vi "LoadRIOSettings.vi"(8 "Error in":errorcluster, 10 "Current ExpState IN":T1={"error"={"status"=FALSE, "code"=0, "source"=""}, "Digitizer DAQmx Tasks"={"TaskArray"=[]}, "DAQ Settings"={"Channel Settings"=[], "Card Settings"=[]}, "Synchronization Settings"={"Synchronizer 0"="", "source terminal"="", "Synchronizer 1"=""}, "DAQ Data"=[], "Next Shot#"="", "System Message"="", "User Shot Notes"="", "Timing Settings"={"Timing Card Settings"=[], "Timing Channel Settings"=[]}, "Timing Tasks"={"TaskArray"=[]}, "Tree"="", "Time Card/Channels"=[], "DAQ Card/Channels"=[], "Program Version"="", "RIO Settings"={"Channel Settings"=[], "Card Settings"=[]}, "RIO References"={"Reference Array"=[]}, "RIO Data"={"RIO Deleaved Data"=[], "Raw Readout"=[]}, "RIO Card/Channels"=[], "DIO Channels"=0, "DIO Settings"={"DIO Channel Array"=[]}, "Tachometer Controls"={"Tach Calibration folder"=path "Z:/Data/Calibration/Tachometer", "PSU2 charging Voltage [kV]"=0.0, "PSU2 Counter"="", "PSU2 task"="PSU2", "PSU3 Counter"="", "PSU3 task"="", "PSU3 charging Voltage [kV]"=0.0}, "Global Settings"={"Initial Background Values"={"Reference Shot #"=0.0, "Background pressure [Torr]"=0.0, "Cryo temp [V]"=0.0, "Cryo temp [K]"=0.0, "Cryotemp Calibration File"=path ""}, "Gas Puffing"={"Gas A type"="N", "Gas B type"="N", "Gas C type"="N", "Gas A pressure [psi]"=0.0, "Gas B pressure [psi]"=0.0, "Gas C pressure [psi]"=0.0, "Innner Electrode"="", "Middle Electrode"="", "Outer Electrode"="", "Gas A bottle pressure [psi]"=0.0, "Gas B bottle pressure [psi]"=0.0, "Gas C bottle pressure [psi]"=0.0}, "PSU Voltages"={"Bias1 Voltage [V]"=0.0, "Bias2 Voltage [V]"=0.0, "PSU1 Voltage [V]"=0.0, "Puff-PSU1 CH1 Voltage [V]"=0.0, "Puff-PSU1 CH2 Voltage [V]"=0.0, "Puff-PSU1 CH3 Voltage [V]"=0.0}, "Scope Details"={"CH1"="", "CH2"="", "CH3"="", "CH4"="", "CH1 Ground State"="Grounded", "CH2 Ground State"="Grounded", "CH3 Ground State"="Grounded", "CH4 Ground State"="Grounded"}}, "Calibrations"={"CryoTemp"={"Comment"="", "X"=[], "Y"=[]}, "PSU2 Tach"={"Comment"="", "X"=[], "Y"=[]}, "PSU3 Tach"={"Comment"="", "X"=[], "Y"=[]}}} {"Global Settings"."Initial Background Values"."Cryo temp [K]" format="%#_4g"; "RIO Settings"."Card Settings"."Sample Rate" format="%#_3p"; "Timing Settings"."Timing Channel Settings"."FrontPanelTime" format="%.3p"; "Timing Settings"."Timing Channel Settings"."Pulse width (s)" format="%.3p"; "Timing Settings"."Timing Channel Settings"."Delay (s)" format="%.3p"; "DAQ Settings"."Card Settings"."Global Edge Type" items=["Rising"=10280, "Falling"=10171]; "DAQ Settings"."Card Settings"."Sample Rate" format="%#_3p"}, 11 "Tree DVR in":refnum<data-value>) -> (0 "Error out":errorcluster, 3 "RIO Settings":T8 {"Card Settings"."Sample Rate" format="%#_3p"})   [LabVIEW 2014]
uses:
  Controls/RIOSettingsExperimentStateCluster.ctl
  Controls/RIOChannelSettingsArrayExperimentStateCluster.ctl
  Controls/RIOSettingsChannelSettings.ctl
  Controls/RIOSettingsCardSettingsArray.ctl
  Controls/RIOSettingsCardSettings.ctl
  <vilib>/userdefined/High Color/nirio_resource_hc.ctl
  <vilib>/MDSplus/Classes/Tree_Class/Tree.lvclass
  Controls/ExperimentStateCluster.ctl
  Controls/DigitizerSettingsChannelSettings.ctl
  Controls/DigitizerSettingsCardSettingsArray.ctl
  Controls/DigitizerSettingsCardSettings.ctl
  Controls/TimingSettings.ctl
  Controls/TimingCardSettings.ctl
  Controls/TimingChannelSettings.ctl
  Controls/RIOData.ctl
  Controls/DIOChannel.ctl
  Controls/TachometerControls.ctl
  Controls/Global Settings/GlobalSettings.ctl
  Controls/Global Settings/InitialBackgroundValues.ctl
  Controls/Global Settings/GasPuffing.ctl
  Controls/Global Settings/PSUVoltages.ctl
  Controls/Global Settings/ScopeDetails.ctl
  Controls/Calibrations/Calibrations.ctl
  Controls/Calibrations/CryoTemoCalibration.ctl
  Controls/Calibrations/PSU2TachCalibration.ctl
  Controls/Calibrations/PSU3TachCalibration.ctl
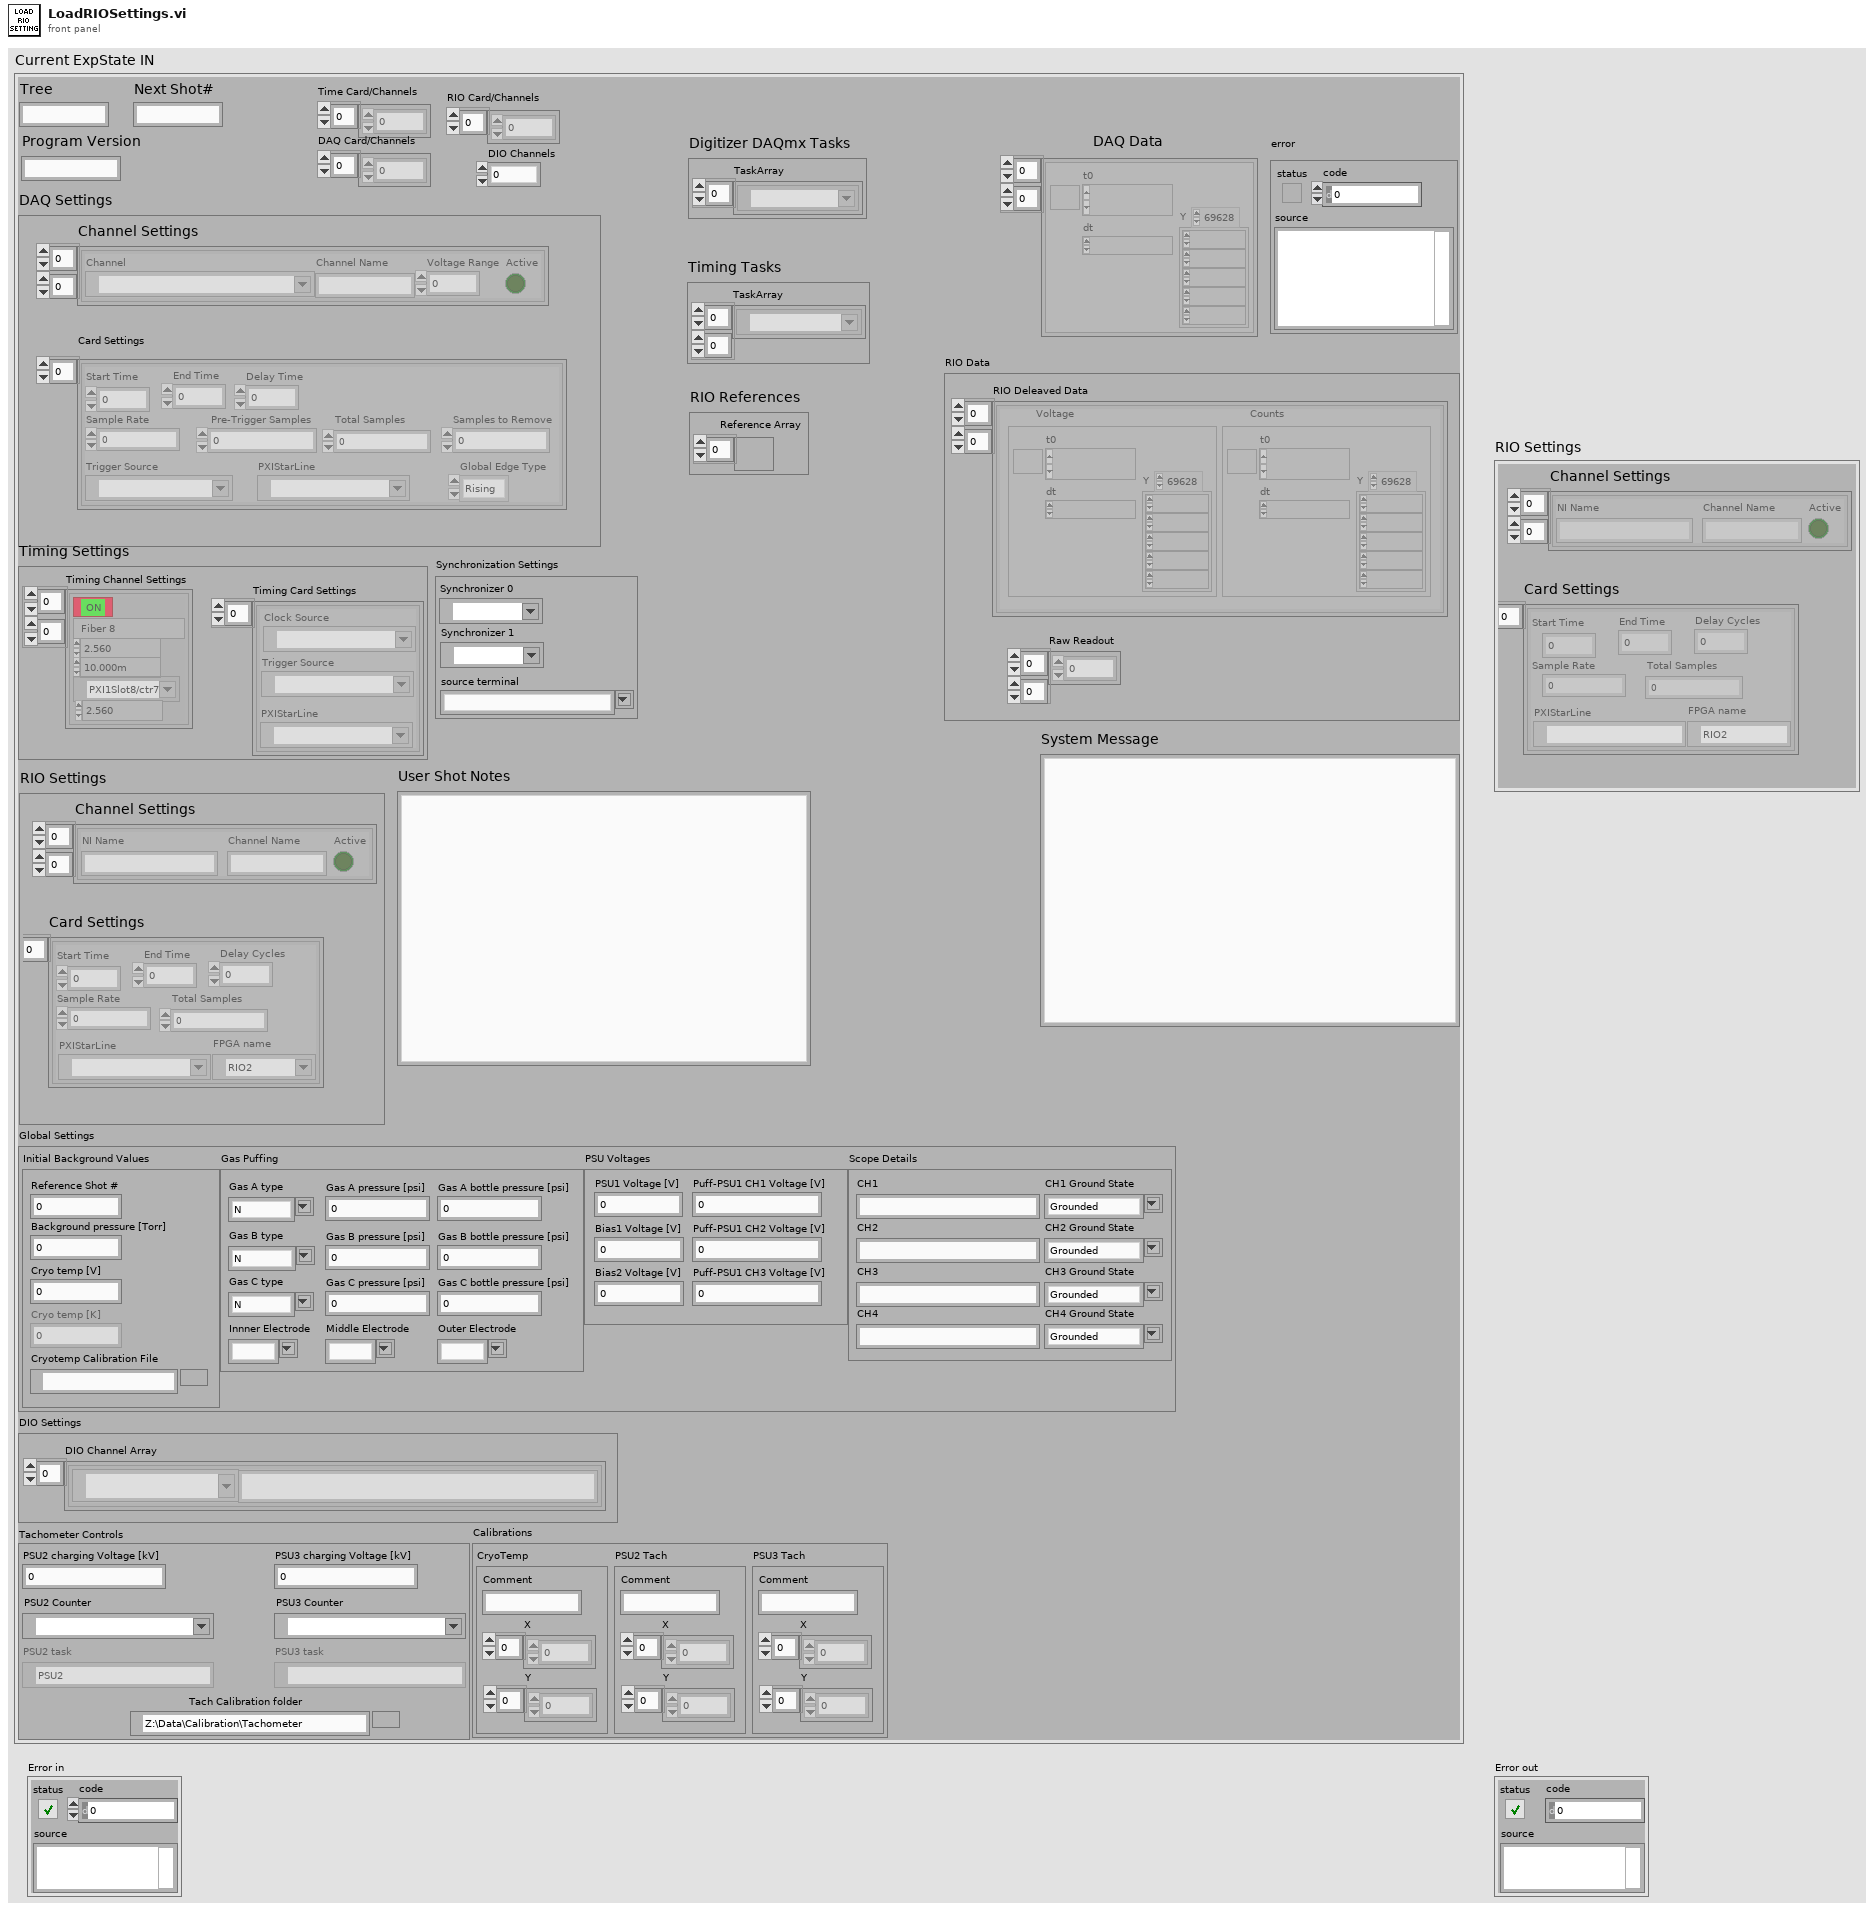
[diagram p1: front panel]
types:
  T1 = typedef "ExperimentStateCluster.ctl" = cluster{"error":errorcluster, "Digitizer DAQmx Tasks":cluster{"TaskArray":refnum<k21>[]}, "DAQ Settings":cluster{"Channel Settings":T2[][], "Card Settings":T3}, "Synchronization Settings":cluster{"Synchronizer 0":refnum<k15>, "source terminal":string, "Synchronizer 1":refnum<k15>}, "DAQ Data":waveform(dbl)[][], "Next Shot#":string, "System Message":string, "User Shot Notes":string, "Timing Settings":T5, "Timing Tasks":cluster{"TaskArray":refnum<k21>[][]}, "Tree":string, "Time Card/Channels":i32[], "DAQ Card/Channels":i32[], "Program Version":string, "RIO Settings":T8, "RIO References":cluster{"Reference Array":refnum<k20>[]}, "RIO Data":T14, "RIO Card/Channels":i32[], "DIO Channels":i32, "DIO Settings":cluster{"DIO Channel Array":T15[]}, "Tachometer Controls":T16, "Global Settings":T17, "Calibrations":T22}
  T2 = typedef "DigitizerSettingsChannelSettings.ctl" = cluster{"Channel":tag, "Channel Name":string, "Voltage Range":dbl, "Active":bool}
  T3 = typedef "DigitizerSettingsCardSettingsArray.ctl" = T4[]
  T4 = typedef "DigitizerSettingsCardSettings.ctl" = cluster{"Start Time":dbl, "End Time":dbl, "Sample Rate":dbl, " Pre-Trigger Samples":u32, "Total Samples":i32, "Samples to Remove":u32, "Trigger Source":tag, "Global Edge Type":i32, "PXIStarLine":tag, "Delay Time":dbl}
  T5 = typedef "TimingSettings.ctl" = cluster{"Timing Card Settings":T6[], "Timing Channel Settings":T7[][]}
  T6 = typedef "TimingCardSettings.ctl" = cluster{"Trigger Source":tag, "Clock Source":tag, "PXIStarLine":tag}
  T7 = typedef "TimingChannelSettings.ctl" = cluster{"Delay (s)":dbl, "Pulse width (s)":dbl, "Active":bool, "Channel Name":string, "counter":tag, "FrontPanelTime":dbl}
  T8 = typedef "RIOSettingsExperimentStateCluster.ctl" = cluster{"Channel Settings":T9, "Card Settings":T11}
  T9 = typedef "RIOChannelSettingsArrayExperimentStateCluster.ctl" = T10[][]
  T10 = typedef "RIOSettingsChannelSettings.ctl" = cluster{"Channel Name":string, "Active":bool, "NI Name":string}
  T11 = typedef "RIOSettingsCardSettingsArray.ctl" = T12[]
  T12 = typedef "RIOSettingsCardSettings.ctl" = cluster{"Start Time":dbl, "End Time":dbl, "Sample Rate":dbl, "Total Samples":u64, "PXIStarLine":tag, "Delay Cycles":u64, "FPGA name":T13}
  T13 = typedef "nirio_resource_hc.ctl" = tag
  T14 = typedef "RIOData.ctl" = cluster{"RIO Deleaved Data":cluster{"Voltage":waveform(dbl), "Counts":waveform(i16)}[][], "Raw Readout":u64[][]}
  T15 = typedef "DIOChannel.ctl" = cluster{"Channel Name":string, "NI Name":tag}
  T16 = typedef "TachometerControls.ctl" = cluster{"Tach Calibration folder":path, "PSU2 charging Voltage [kV]":dbl, "PSU2 Counter":tag, "PSU2 task":refnum<k21>, "PSU3 Counter":tag, "PSU3 task":refnum<k21>, "PSU3 charging Voltage [kV]":dbl}
  T17 = typedef "GlobalSettings.ctl" = cluster{"Initial Background Values":T18, "Gas Puffing":T19, "PSU Voltages":T20, "Scope Details":T21}
  T18 = typedef "InitialBackgroundValues.ctl" = cluster{"Reference Shot #":dbl, "Background pressure [Torr]":dbl, "Cryo temp [V]":dbl, "Cryo temp [K]":dbl, "Cryotemp Calibration File":path}
  T19 = typedef "GasPuffing.ctl" = cluster{"Gas A type":string, "Gas B type":string, "Gas C type":string, "Gas A pressure [psi]":dbl, "Gas B pressure [psi]":dbl, "Gas C pressure [psi]":dbl, "Innner Electrode":string, "Middle Electrode":string, "Outer Electrode":string, "Gas A bottle pressure [psi]":dbl, "Gas B bottle pressure [psi]":dbl, "Gas C bottle pressure [psi]":dbl}
  T20 = typedef "PSUVoltages.ctl" = cluster{"Bias1 Voltage [V]":dbl, "Bias2 Voltage [V]":dbl, "PSU1 Voltage [V]":dbl, "Puff-PSU1 CH1 Voltage [V]":dbl, "Puff-PSU1 CH2 Voltage [V]":dbl, "Puff-PSU1 CH3 Voltage [V]":dbl}
  T21 = typedef "ScopeDetails.ctl" = cluster{"CH1":string, "CH2":string, "CH3":string, "CH4":string, "CH1 Ground State":string, "CH2 Ground State":string, "CH3 Ground State":string, "CH4 Ground State":string}
  T22 = typedef "Calibrations.ctl" = cluster{"CryoTemp":T23, "PSU2 Tach":T24, "PSU3 Tach":T25}
  T23 = typedef "CryoTemoCalibration.ctl" = cluster{"Comment":string, "X":dbl[], "Y":dbl[]}
  T24 = typedef "PSU2TachCalibration.ctl" = cluster{"Comment":string, "X":dbl[], "Y":dbl[]}
  T25 = typedef "PSU3TachCalibration.ctl" = cluster{"Comment":string, "X":dbl[], "Y":dbl[]}
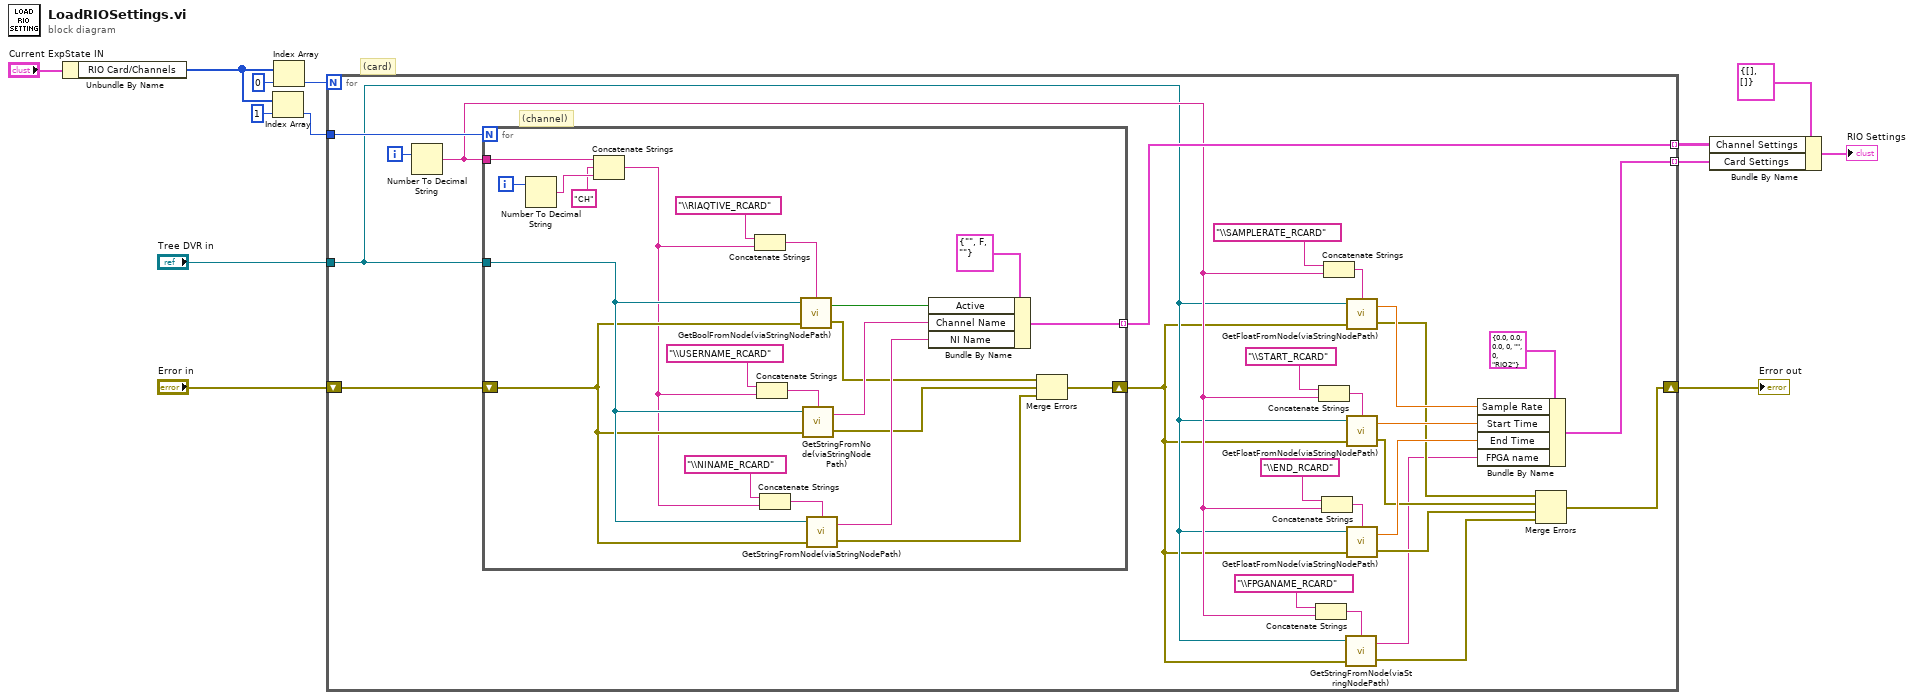
[diagram p0: block diagram]
diagram:
  # "(card)"
  n1 = Unbundle By Name("Current ExpState IN") -> ("RIO Card/Channels"=w7:i32[])
  n2 = Index Array(array=w7, index=1) -> (element=w5:i32)
  n3 = Index Array(array=w7, index=0) -> (element=w6:i32)
  n4 = for {
    N: w6 -> [_]
    shift-right: [w22] -> w11
    shift-left: "Error in" -> [w37]
    tunnel: w5 -> [w38]
    tunnel: "Tree DVR in" -> [w18]
    tunnel: [w36] -> w4 mode=indexing
    tunnel: [w26] -> w3 mode=indexing
    i -> [w39]
    # "(channel)"
    n5 = Number To Decimal String(number=w39) -> (decimal integer string=w20:string)  [unwired: 1 in]
    n6 = for {
      N: w38 -> [_]
      tunnel: w20 -> [w60]
      tunnel: w18 -> [w54]
      shift-right: [w42] -> w17
      shift-left: w37 -> [w53]
      tunnel: [w41] -> w36 mode=indexing
      i -> [w61]
      n7 = Number To Decimal String(number=w61) -> (decimal integer string=w59:string)  [unwired: 1 in]
      n8 = Concatenate Strings(w60, "CH" ("string"), w59) -> (w48:string)
      n9 = Concatenate Strings("\\RIAQTIVE_RCARD" ("string"), w48) -> (w56:string)
      n10 = Concatenate Strings("\\USERNAME_RCARD" ("string"), w48) -> (w51:string)
      n11 = Concatenate Strings("\\NINAME_RCARD" ("string"), w48) -> (w47:string)
      n12 = call "GetBoolFromNode(viaStringNodePath).vi"("Path"=w56, "error in"=w53, "Tree DVR in"=w54) -> ("error out"=w45:errorcluster, "Bool Out"=w55:bool)  [unwired: 1 in]
      n13 = call "GetStringFromNode(viaStringNodePath).vi"("Path"=w51, "error in"=w53, "Tree DVR in"=w54) -> ("error out"=w44:errorcluster, "String out"=w50:string)  [unwired: 1 in]
      n14 = call "GetStringFromNode(viaStringNodePath).vi"("Path"=w47, "error in"=w53, "Tree DVR in"=w54) -> ("error out"=w43:errorcluster, "String out"=w46:string)  [unwired: 1 in]
      n15 = Bundle By Name(cluster=T10 {"Channel Name"="", "Active"=FALSE, "NI Name"=""} ("Channel Setting"), "Active"=w55, "Channel Name"=w50, "NI Name"=w46) -> (w41:T10)
      n16 = Merge Errors(w45, w44, w43) -> (w42:errorcluster)
    }
    n17 = Concatenate Strings("\\FPGANAME_RCARD" ("string"), w20) -> (w19:string)
    n18 = Concatenate Strings("\\START_RCARD" ("string"), w20) -> (w32:string)
    n19 = Concatenate Strings("\\END_RCARD" ("string"), w20) -> (w30:string)
    n20 = Concatenate Strings("\\SAMPLERATE_RCARD" ("string"), w20) -> (w34:string)
    n21 = call "GetStringFromNode(viaStringNodePath).vi"("Path"=w19, "error in"=w17, "Tree DVR in"=w18) -> ("error out"=w16:errorcluster, "String out"=w14:string)  [unwired: 1 in]
    n22 = call "GetFloatFromNode(viaStringNodePath).vi"("Path"=w34, "error in"=w17, "Tree DVR in"=w18) -> ("error out"=w25:errorcluster, "Float64"=w29:dbl)  [unwired: 1 in]
    n23 = call "GetFloatFromNode(viaStringNodePath).vi"("Path"=w32, "error in"=w17, "Tree DVR in"=w18) -> ("error out"=w24:errorcluster, "Float64"=w27:dbl)  [unwired: 1 in]
    n24 = call "GetFloatFromNode(viaStringNodePath).vi"("Path"=w30, "error in"=w17, "Tree DVR in"=w18) -> ("error out"=w23:errorcluster, "Float64"=w28:dbl)  [unwired: 1 in]
    n25 = Bundle By Name(cluster=T12 {"Start Time"=0.0, "End Time"=0.0, "Sample Rate"=0.0, "Total Samples"=0, "PXIStarLine"="", "Delay Cycles"=0, "FPGA name"="RIO2"} ("Card Setting"), "Sample Rate"=w29, "Start Time"=w27, "End Time"=w28, "FPGA name"=w14) -> (w26:T12)
    n26 = Merge Errors(w25, w24, w23, w16) -> (w22:errorcluster)
  }
  "Error out" <- w11
  n27 = Bundle By Name(cluster=T8 {"Channel Settings"=[], "Card Settings"=[]} ("RIO Settings"), "Channel Settings"=w4, "Card Settings"=w3) -> (→"RIO Settings":T8)
